vi "WriteI32.vi"(0 "ObjHandle in":T1, 1 "功能选择":u16(ring)=24672 items=["rwCtrlWordU16"=24640, "rStatusWordU16"=24641, "rwVlTgtVelU16"=24642, "rVlVelDemU16"=24643, "rwOperationModeI8"=24672, "rOperationModeI8"=24673, "rPosDemI32"=24674, "rPosAct*I32"=24675, "rPosActI32"=24676, "rVelSenActI32"=24681, "rVelDemI32"=24683, "rwTorqTgt"=24689, "rwTorqMaxU16"=24690, "rTorqDemI16"=24692, "rTorqActI16"=24695, "rwPosTgtI32"=24698, "rwMaxMotorSpdU32"=24704, "rwPrfVelU32"=24705, "rwPrfAccU32"=24707, "rwPrfDeaccU32"=24708, "rwTorqSlopeU32"=24711, "rTorqPrfTypeI16"=24712, "rwHomMethI8"=24728, "rwHomSpdU32"=24729, "rwTgtVelI32"=24831], 2 "Data":i32, 3 "error in":errorcluster, 4 "Sub Index":u8 format="%.0x") -> (5 "写入数组":u8[](array[numeric]) format="%x", 7 "ObjHandle out":T1, 8 "Data":u32, 10 "Error out":errorcluster {"code" format="%.0x"})   [LabVIEW 2019]
uses:
  <vilib>/nican/nican.llb/xobjhandle.ctl
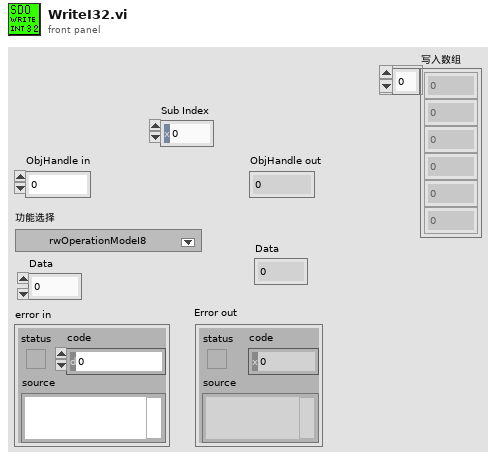
[diagram p1: front panel]
types:
  T1 = typedef "xobjhandle.ctl" = u32
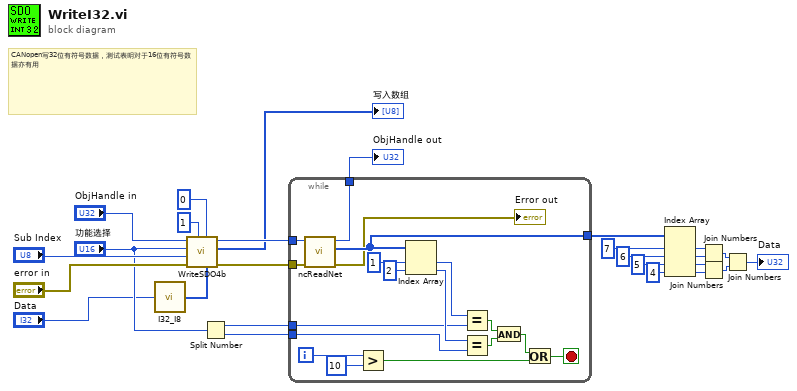
[diagram p0: block diagram]
diagram:
  # "CANopen写32位有符号数据，测试表明对于16位有符号数据亦有用"
  n1 = call "I32_I8.vi"("x"="Data") -> ("数组"=w3:i8[])  [unwired: 4 in]
  n2 = call "WriteSDO4b.vi"("data array"=w3, "R/W"=u8 0, "Node ID"=u8 1, "error in"="error in", "Sub Index"="Sub Index", "Index"="功能选择", "ObjHandle in"="ObjHandle in") -> ("error out"=w8:errorcluster, "写入数组"=→"写入数组":u8[], "ObjHandle out"=w10:T1)  [unwired: 2 in]
  n3 = Split Number(x="功能选择") -> (hi(x)=w7:u8, lo(x)=w6:u8)
  n4 = while {
    tunnel: w10 -> [w44]
    tunnel: [w37] -> w22
    tunnel: w8 -> [w36]
    tunnel: [w35] -> w9
    tunnel: w7 -> [w32]
    tunnel: w6 -> [w31]
    i -> [w43]
    stop <- w39 stop-if-true
    n5 = call <vilib>:"ncReadNet.vi"("ObjHandle in"=w44, "Error in"=w36) -> ("ObjHandle out"=w35:T1, "Data"=w37:u8[], "Error out"=→"Error out":errorcluster)  [unwired: 2 in, 4 out]
    n6 = Greater?(x=w43, y=10) -> (0:w38:bool)
    n7 = Index Array(array=w37, index #1=1 ("索引"), index #2=2 ("索引")) -> (element #1=w40:u8, element #2=w33:u8)
    n8 = Equal?(x=w40, y=w32) -> (x = y?=w30:bool)
    n9 = Equal?(x=w33, y=w31) -> (x = y?=w29:bool)
    n10 = And(x=w30, y=w29) -> (x .and. y?=w28:bool)
    n11 = Or(x=w28, y=w38) -> (x .or. y?=w39:bool)
  }
  "ObjHandle out" <- w9
  n12 = Index Array(array=w22, index #1=7 ("索引"), index #2=6 ("索引"), index #3=5 ("索引"), index #4=4 ("索引")) -> (element #1=w17:u8, element #2=w16:u8, element #3=w15:u8, element #4=w14:u8)
  n13 = Join Numbers(hi=w17, lo=w16) -> ((hi.lo)=w13:u16)
  n14 = Join Numbers(hi=w15, lo=w14) -> ((hi.lo)=w12:u16)
  n15 = Join Numbers(hi=w13, lo=w12) -> ((hi.lo)=→"Data":u32)
